vi "Start.vi"(8 "ErrorIn":errorcluster, 11 "OpenCVCamIn":refnum<class "OpenCVCam.lvclass">) -> (0 "ErrorOut":errorcluster, 3 "OpenCVCamOut":refnum<class "OpenCVCam.lvclass">)   [LabVIEW 2021, in "OpenCVCam.lvclass"]
uses:
  OpenCVCam.lvclass
  C:/Localdata/Projects/TriekselSoft/TriekselsoftApplicationFramework/Source/.Externals/Library_YAF/YActor/YActor.lvclass
  Library_YAF/YActor/YActor.lvclass/YActor.ctl
  Library_YAF/YActor/ExeCmd_sync.vi
  Library_YAF/YActor/private/SendCommand.vi
  Library_YAF/YActor/private/WaitForReply.vi
  Library_YAF/YActor/private/CreateLocalVI.vi
  Library_YAF/YActor/private/ExeuteInlineVI.vi
  Library_YAF/YActor/private/GetRemoteVIRef.vi
  Library_YAF/YActor/private/GetNameOfVI.vi
  Library_YAF/YActor/QuickCast.vi
  Library_YAF/YActor/private/VINameProperty.vi
  Library_YAF/YActor/private/MessageCounter.vi
  Library_YAF/YActor/InlineReferencePool.vi
  Library_YAF/YActor/private/ExecuteVI.vi
  Library_YAF/YActor/YActor.lvclass
  C:/Localdata/Projects/TriekselSoft/TriekselsoftApplicationFramework/Source/.Externals/Library_YAF/YAFTAF/YAFTAF.lvclass
  C:/Localdata/Projects/TriekselSoft/TriekselsoftApplicationFramework/Source/.Externals/Interface_UserInterface_IFrontPanel/IFrontPanel/IFrontPanel.lvclass
  C:/Localdata/Projects/TriekselSoft/TriekselsoftApplicationFramework/Source/.Externals/Interface_TAF_IInterface/IInterface/IInterface.lvclass
  C:/Localdata/Projects/TriekselSoft/TriekselsoftApplicationFramework/Source/.Externals/Interface_Object_ICreateDestroy/ICreateDestroy/ICreateDestroy.lvclass
  C:/Localdata/Projects/TriekselSoft/TriekselsoftApplicationFramework/Source/.Externals/Interface_Object_IPersistentData/IPersistentData/IPersistentData.lvclass
  C:/Localdata/Projects/TriekselSoft/TriekselsoftApplicationFramework/Source/.Externals/Interface_TAF_ITAFObject/ITAFObject/ITAFObject.lvclass
  C:/Localdata/Projects/TriekselSoft/TriekselsoftApplicationFramework/Source/.Externals/YAFTAFModule_OpenCV_Camera/OpenCVCam/OpenCVCam.lvclass
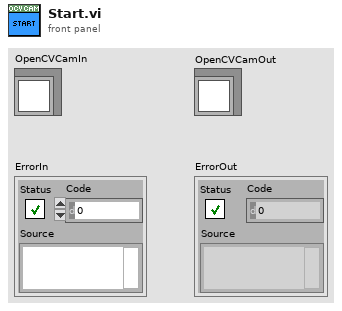
[diagram p1: front panel]
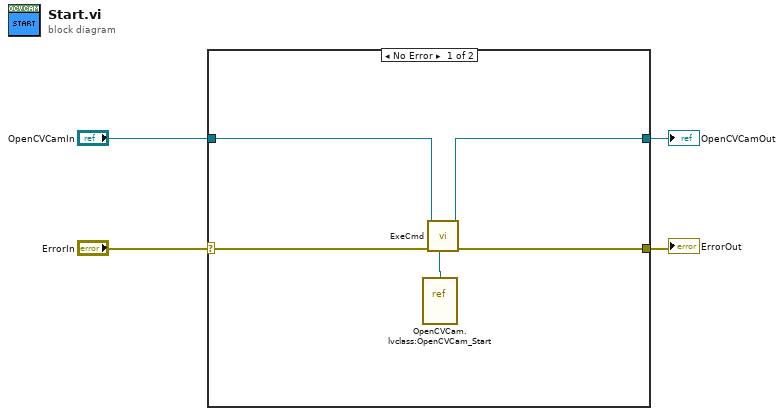
[diagram p0: block diagram]
diagram:
  n1 = case shown="No Error" "ErrorIn" {
    selector: "ErrorIn" -> [w9 w11]
    tunnel: [w8 w11] -> w3
    tunnel: [w5 w10] -> w1
    tunnel: "OpenCVCamIn" -> [w6 w10]
    frame No Error {
      n2 = vi-ref "OpenCVCam.lvclass:OpenCVCam_Start.vi"() -> (w7:refnum<vi>)
      n3 = call-poly "ExeCmd.vi"("CmdVIRef"=w7, "ErrorIn"=w9, "YActorIn"=w6) -> ("ErrorOut"=w8:errorcluster, "YActorOut"=w5:refnum<class "OpenCVCam.lvclass">)  [unwired: 6 in, 1 out]
    }
    frame Error {
    }
  }
  "ErrorOut" <- w3
  "OpenCVCamOut" <- w1
